vi "Get.vi"(8 "error in (no error)":errorcluster, 11 "Template":refnum<class "Singleton.lvclass">) -> (0 "error out":errorcluster, 3 "object":refnum<class "Singleton.lvclass">)   [LabVIEW 2014, in "Singleton.lvlib" / "Singleton.lvclass"]
uses:
  Singleton.lvclass
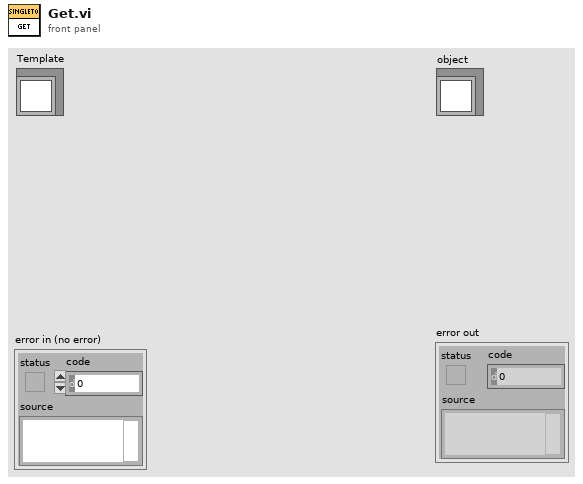
[diagram p1: front panel]
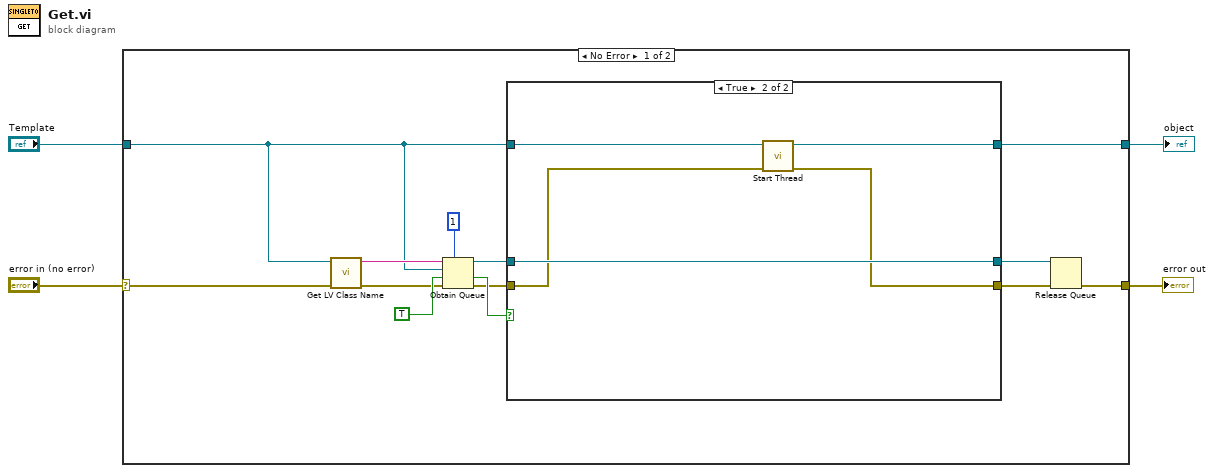
[diagram p0: block diagram]
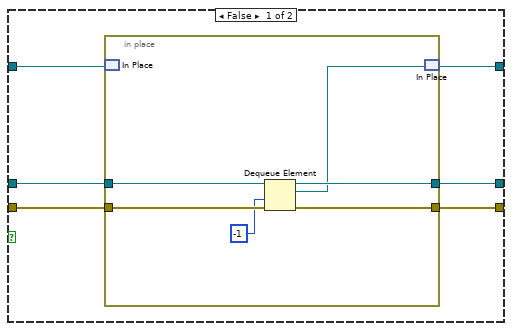
[diagram p2: hidden frame]
diagram:
  n1 = case shown="No Error" "error in (no error)" {
    selector: "error in (no error)" -> [w14 w36]
    tunnel: [w5 w36] -> w3
    tunnel: "Template" -> [w6 w35]
    tunnel: [w7 w35] -> w1
    frame No Error {
      n2 = call <vilib>:"Get LV Class Name.vi"("error in (no error)"=w14, "object"=w6) -> ("error out"=w13:errorcluster, "class name"=w17:string)  [unwired: 8 in]
      n3 = Obtain Queue(max queue size (-1, unlimited)=1, name (unnamed)=w17, element data type=w6, create if not found? (T)=TRUE, error in (no error)=w13) -> (queue out=w10:refnum<queue>, created new?=w12:bool, error out=w11:errorcluster)
      n4 = case shown="True" w12 {
        tunnel: w11 -> [w22 w31]
        tunnel: w10 -> [w23 w34]
        tunnel: [w18 w33] -> w7
        tunnel: [w21 w32] -> w9
        tunnel: w6 -> [w19 w30]
        tunnel: [w20 w34] -> w8
        frame False {
          n5 = in-place {
            in-place-border: w23 -> [w29]
            in-place-border: w22 -> [w28]
            in-place-border: [w27] -> w21
            in-place-border: [w26] -> w20
            n6 = in-place-match #1(w19) -> ()  [unwired: 1 out]
            n7 = Dequeue Element(queue=w29, timeout in ms (-1)=-1, error in (no error)=w28) -> (queue out=w26:refnum<queue>, element=w24:refnum<class "Singleton.lvclass">, error out=w27:errorcluster)  [unwired: 1 out]
            n8 = in-place-match #1(w24) -> (w18:refnum<class "Singleton.lvclass">)
          }
        }
        frame True {
          n9 = call "Start Thread.vi"("error in (no error)"=w31, "Template"=w30) -> ("error out"=w32:errorcluster, "object"=w33:refnum<class "Singleton.lvclass">)  [unwired: 8 in]
        }
      }
      n10 = Release Queue(queue=w8, error in (no error)=w9) -> (error out=w5:errorcluster)  [unwired: 1 in, 2 out]
    }
    frame Error {
    }
  }
  "error out" <- w3
  "object" <- w1
